vi "MagLab OSF Sync .vi"(8 "error in":errorcluster) -> (0 "error out":errorcluster)   [LabVIEW 2020]
uses:
  Utilities/iCalendar/Extract iCalendar String.ctl
  System.Windows.Forms
panel:
  in  "Password":string
  in  "User portal login":string="fedor@lanl.gov"
  in  "Browse experiment":bool
  in  "Sync to OSF":bool
  in  "Load calendar":bool
  in  "Tab Control":T1(tab)
  in  "User portal":refnum<k24>(container)
  in  "Experiments list":i32(listbox)=-1
  out "IDs":string[](array[string])
  out "Names":string[](array[string])
  in  "Page info":bool
  in  "User portal URL":string="https://users.magnet.fsu.edu/Users/LogIn.aspx"
  in  "Facility Calendar URL":string="https://users.magnet.fsu.edu/Experiments/Calendar.aspx"
  out "Elements count":i32
  out "time lapsed":u32 format="%.0fms"
  in  "OSF Token":string
  out "Selected experiment":T2
  out "Experiments":T2[](array[typedef])
  out "Wiki ID":string
  in  "Stop Button":bool
  # "users.magnet.fsu.edu/Experiments/Calendar.aspx?facilityID=5&MagnetSystemID=54"
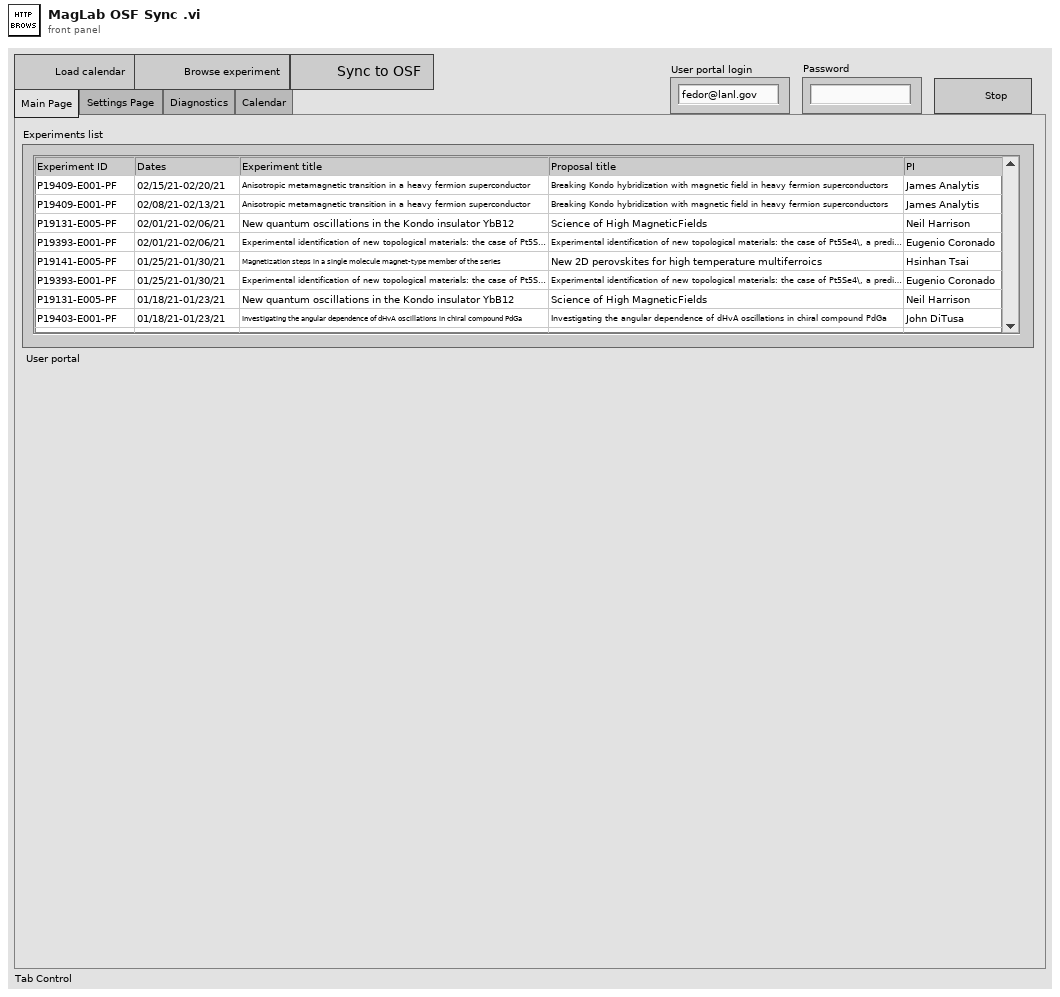
[diagram p1: front panel]
types:
  T1 = enum32{"Main Page", "Settings Page ", "Diagnostics", "Calendar"}
  T2 = typedef "Extract iCalendar String.ctl" = cluster{"Orginizer Name":string, "Location":string, "Summary":string, "Start Date and Time":timestamp, "End Date and Time":timestamp, "Description":string, "Proposal title":string, "Experiment":string, "URL":string, "Experiment title":string, "PI":string, "Proposal":string}
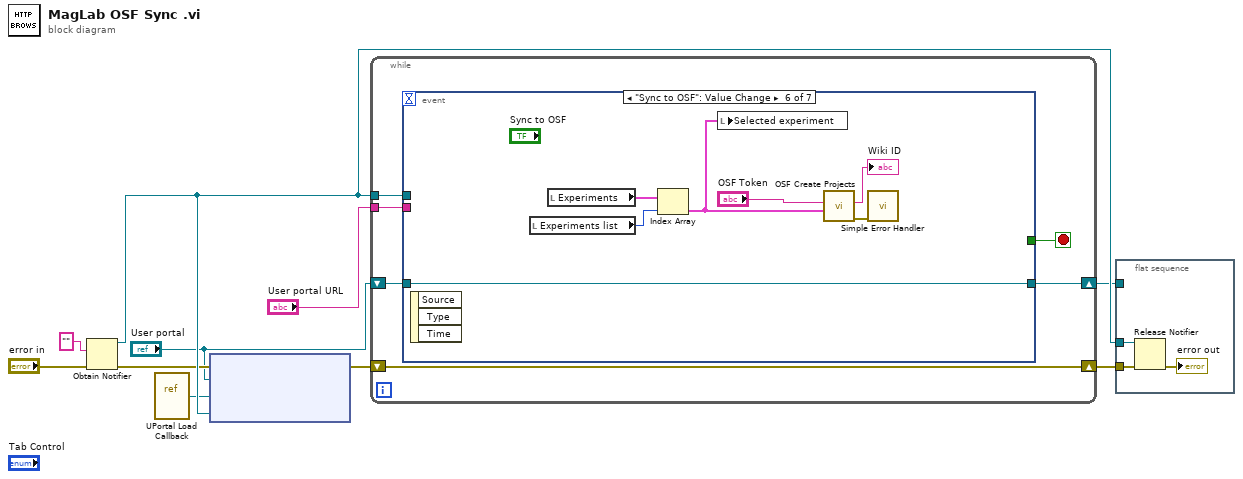
[diagram p0: block diagram]
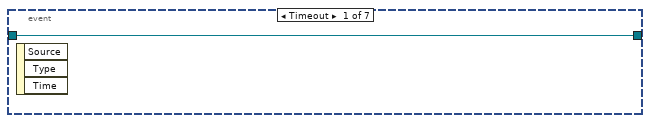
[diagram p2: hidden frame]
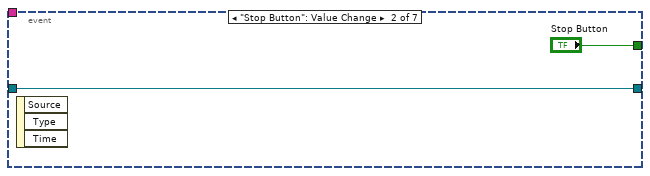
[diagram p3: hidden frame]
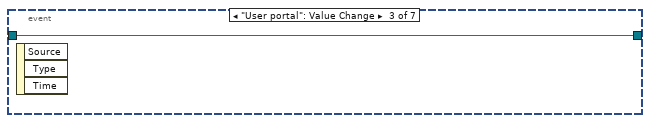
[diagram p4: hidden frame]
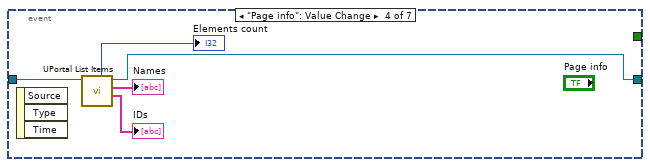
[diagram p5: hidden frame]
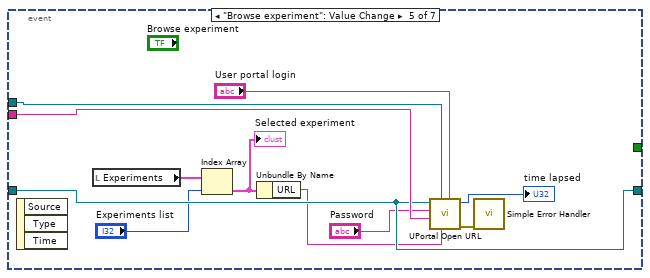
[diagram p6: hidden frame]
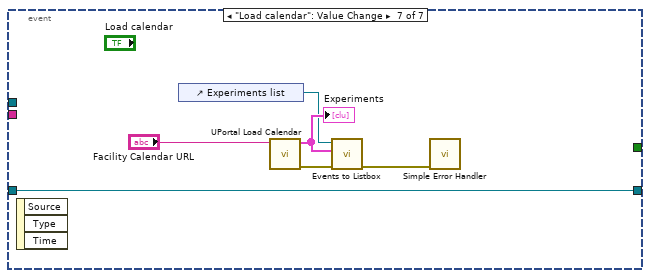
[diagram p7: hidden frame]
diagram:
  n1 = Obtain Notifier(notification data type="", error in (no error)="error in") -> (notifier out=w7:refnum<notifier>, error out=w5:errorcluster)  [unwired: 2 in, 1 out]
  n2 = vi-ref "UPortal Load Callback.vi"() -> ("vi reference"=w6:refnum<vi>)
  n3 = node(w5, "User portal", w6, w7) -> (w2:errorcluster)  [unwired: 1 in, 1 out]
  n4 = while {
    shift-right: [w14] -> w3
    shift-left: "User portal" -> [w15]
    tunnel: "User portal URL" -> [w13]
    tunnel: w7 -> [w12]
    shift-right: [w11] -> w1
    shift-left: w2 -> [w11]
    stop <- w16 stop-if-true
    n5 = event shown="[5] \"Sync to OSF\": Value Change" {
      selector: _ -> [_ _ _ _ _ _ _]
      dyn-events: _ -> [_ _ _ _ _ _ _]
      timeout: _ -> [_ _ _ _ _ _ _]
      tunnel: [_ "Stop Button" _ _ _ _ _] -> w16
      tunnel: w15 -> [w17 w18 w20 w22 w32 w41 w48]
      tunnel: [w17 w18 w20 w21 w32 w41 w48] -> w14
      tunnel: w13 -> [_ _ _ _ w36 _ _]
      tunnel: w12 -> [_ _ _ _ w34 _ _]
      event Timeout {
        n6 = event-data() -> ()  [unwired: 1 in, 3 out]
      }
      event "Stop Button": Value Change {
        n7 = event-data() -> ()  [unwired: 1 in, 3 out]
      }
      event "User portal": Value Change {
        n8 = event-data() -> ()  [unwired: 1 in, 3 out]
      }
      event "Page info": Value Change {
        n9 = event-data() -> ()  [unwired: 1 in, 3 out]
        n10 = call "UPortal List Items.vi"(".NET Refnum in"=w22) -> ("Array"=→"IDs":string[], "Array 2"=→"Names":string[], ".NET Refnum out"=w21:refnum<k24>, "Count"=→"Elements count":i32)  [unwired: 6 in, 1 out]
      }
      event "Browse experiment": Value Change {
        n11 = event-data() -> ()  [unwired: 1 in, 3 out]
        n12 = local read "Experiments"() -> (w29:T2[])
        n13 = Index Array(array=w29, index="Experiments list") -> (element=w26:T2)
        "Selected experiment" <- w26
        n14 = Unbundle By Name(w26) -> ("URL"=w27:string)
        n15 = call "UPortal Open URL.vi"("MagLab User Name"="User portal login", "URL"=w27, "notifier in"=w34, "User portal URL"=w36, "Password"="Password", ".NET Refnum in"=w32) -> ("error out"=w35:errorcluster, "time lapsed"=→"time lapsed":u32)  [unwired: 4 in]
        n16 = call <vilib>:"Simple Error Handler.vi"("error in (no error)"=w35) -> ()  [unwired: 4 in, 5 out]
      }
      event "Sync to OSF": Value Change {
        n17 = event-data() -> ()  [unwired: 1 in, 3 out]
        n18 = local read "Experiments list"() -> (w39:i32)
        n19 = local read "Experiments"() -> (w38:T2[])
        n20 = Index Array(array=w38, index=w39) -> (element=w37:T2)
        n21 = local write "Selected experiment"(w37) -> ()
        n22 = call "OSF Create Projects.vi"("Proposal Data"=w37, "Token"="OSF Token") -> ("error out"=w40:errorcluster, "Wiki ID"=→"Wiki ID":string)  [unwired: 8 in]
        n23 = call <vilib>:"Simple Error Handler.vi"("error in (no error)"=w40) -> ()  [unwired: 4 in, 5 out]
      }
      event "Load calendar": Value Change {
        n24 = event-data() -> ()  [unwired: 1 in, 3 out]
        n25 = control-ref of="Experiments list"() -> (w44:refnum<vi>)
        n26 = call "UPortal Load Calendar.vi"("Calendar URL"="Facility Calendar URL") -> ("error out"=w47:errorcluster, "Events out"=w45:T2[])  [unwired: 9 in]
        "Experiments" <- w45
        n27 = call "Events to Listbox.vi"("error in"=w47, "Events"=w45, "Listbox ref"=w44) -> ("error out"=w46:errorcluster)  [unwired: 7 in, 1 out]
        n28 = call <vilib>:"Simple Error Handler.vi"("error in (no error)"=w46) -> ()  [unwired: 4 in, 5 out]
      }
    }
  }
  n29 = flat-sequence {
    tunnel: w7 -> [w51]
    tunnel: w3 -> [_]
    tunnel: w1 -> [w50]
    frame #0 {
      n30 = Release Notifier(notifier=w51, error in (no error)=w50) -> (error out=→"error out":errorcluster)  [unwired: 1 in, 2 out]
    }
  }
